vi "PassInterception.vi"(7 "Ally?":bool, 8 "error in (no error)":errorcluster, 9 "Game":refnum<class "Game.lvclass">, 10 "Point":dbl[](array[numeric]), 11 "object in":refnum<class "Utilities.lvclass">) -> (0 "error out":errorcluster, 2 "Evaluation":dbl, 3 "object out":refnum<class "Utilities.lvclass">)   [LabVIEW 2023, in "Utilities.lvclass"]
uses:
  Utilities.lvclass
  Game_class/Game.lvclass
  Game_class/Game.lvclass/Game.ctl
  Referee_class/Referee.lvclass/Referee.ctl
  Team_class/Team.lvclass/Team.ctl
  Object_class/Object.lvclass/Object.ctl
  Robot_class/Robot.lvclass/Robot.ctl
  <vilib>/Analysis/coordinate.llb/2D Cartesian Coordinate Shift (Scalar).vi
  <vilib>/Analysis/coordinate.llb/2D Cartesian Coordinate Rotation (Scalar).vi
  Robot_class/Read id.vi
  Object_class/Read position(x,y).vi
  Game_class/Read Referee.vi
  Game_class/Read EnemyRef.vi
  Game_class/Read BallRef.vi
  Game_class/Read NewParameters.vi
  Game_class/Read AllyRef.vi
  Team_class/Read RobotRef.vi
  Referee_class/Read enemy_goalie_id.vi
  Referee_class/Read our_goalie_id.vi
  Ally_class/Ally.lvclass
  Ball_class/Ball.lvclass
  Enemy_class/Enemy.lvclass
  Robot_class/Robot.lvclass
  Referee_class/Referee.lvclass
  <vilib>/Analysis/NI_AALPro.lvlib
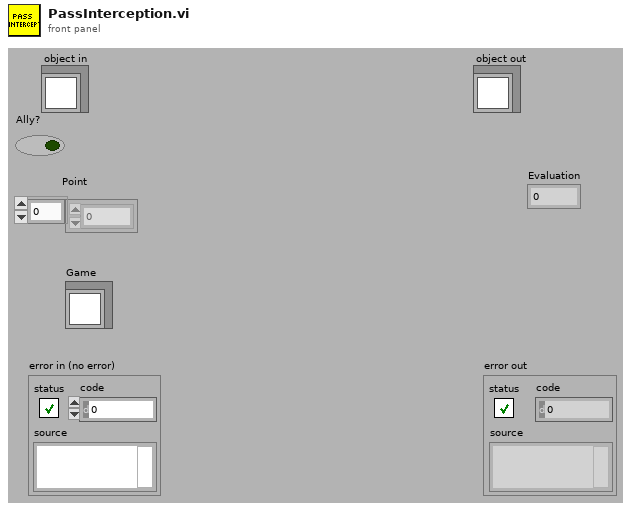
[diagram p1: front panel]
types:
  T1 = typedef "NewParameters.ctl" = cluster{"PenaltyDistance":dbl, "DistanceAttackerToBackBall":dbl, "Division":enum16{"Div B", "Div A"}, "DistanceToAvoidyEnemyRobot":dbl, "BallPlacementDistance":dbl, "DisatanceBehindBallToStealBall":dbl, "MaxDistanceToPositionKickoff":dbl, "BlockEnemyTarget":bool, "MaxStopVAng":dbl, "DistanceMarkerToEnemy":dbl, "IgnoreDribblerContact":bool, "DistanceToBeginEnemyPosession":dbl, "GoToBallWhenEnemyNotMoving":bool, "EnemyDistanceToReduceVelocity":dbl, "TurnOnEnemyDistanceToReduceVelocity":bool, "EnemyDistanceToShootOutBall":dbl, "DefenseKickBall":bool, "MoreKickToGoal? (0-0.3)":dbl, "ChipKickInEnemyField":bool, "ShootOutRobotId":dbl, "FieldLenghtDenominatorInShootOut":dbl, "AdjustPositionInBallPlacement":bool, "PowerGodPass":dbl, "VelocityAbortEnemyPos":dbl, "MaxDistToBeginPass":dbl, "MinDistToBeginPass":dbl, "VelocityInDirects":dbl, "BadDribblerIDs":i32[], "NewKickToDistanceAroundBall":dbl, "PowerAvoidColisionMarker":dbl, "DistanceToAvoidColisionMarker":dbl, "AvoidBallKick":dbl, "DistanceTryKick":dbl, "SuicideKickDIstance":dbl, "AdjustFirstKickDistance":dbl, "AvoidAimLessKick":dbl, "DistanceToAvoidyEnemyShootRobot ":dbl, "NumberOfMarkers":dbl, "PotField":bool, "PIDLateral":bool, "MinDistanceFirstKickX":dbl, "MinDistanceFirstKickY":dbl, "FractionOfDistToTouchGround\nAfterChipKick":dbl, "FractionOfKickxWhen\nComposedWithKickz":dbl, "Style":T2, "MoveInTurnState":bool, "DistFromEnemyToConsider\nMoveInTurnState":dbl, "CascadePID":bool, "TurnAroundParameters":cluster{"Radius":dbl, "Multiplier":dbl, "ChordAngle":dbl}, "SafeDriveVel":dbl, "DistanceToGoToBackBall":dbl, "minDistanceToNotFinishEnemyPossession":dbl, "OneTouchShot":cluster{"angleFactor":dbl, "maxAngle":dbl, "Attack":bool, "Defense":bool}, "OpenAngleToGoal":cluster{"minAngle":dbl, "maxAngle":dbl, "minEvaluation":dbl}, "ShotInterception":cluster{"shotSpeed":dbl, "minEnemySpeed":dbl, "maxEnemySpeed":dbl, "minEvaluation":dbl}, "AllyTeamArray":T3[], "maxDefendersNumber":i32, "Zone":cluster{"GuardPositionArray":dbl[][], "ZoneMidField":dbl[], "CenterForwardWidth":dbl}, "MinEvaluationToShoot":dbl, "PassInterception":cluster{"maxPassSpeed":dbl, "minPassSpeed":dbl, "minEnemySpeed":dbl, "chipPassDistance":dbl, "chipPassEvaluation":dbl, "minEvaluation":dbl, "maxEnemySpeed":dbl}, "PassDistance":cluster{"maxDistance":dbl, "minDistance":dbl}}
  T2 = typedef "Style.ctl" = enum16{"Insanity", "Offensive", "Defensive"}
  T3 = typedef "AllyTeam.ctl" = enum16{"Keeper", "Defender", "Attacker"}
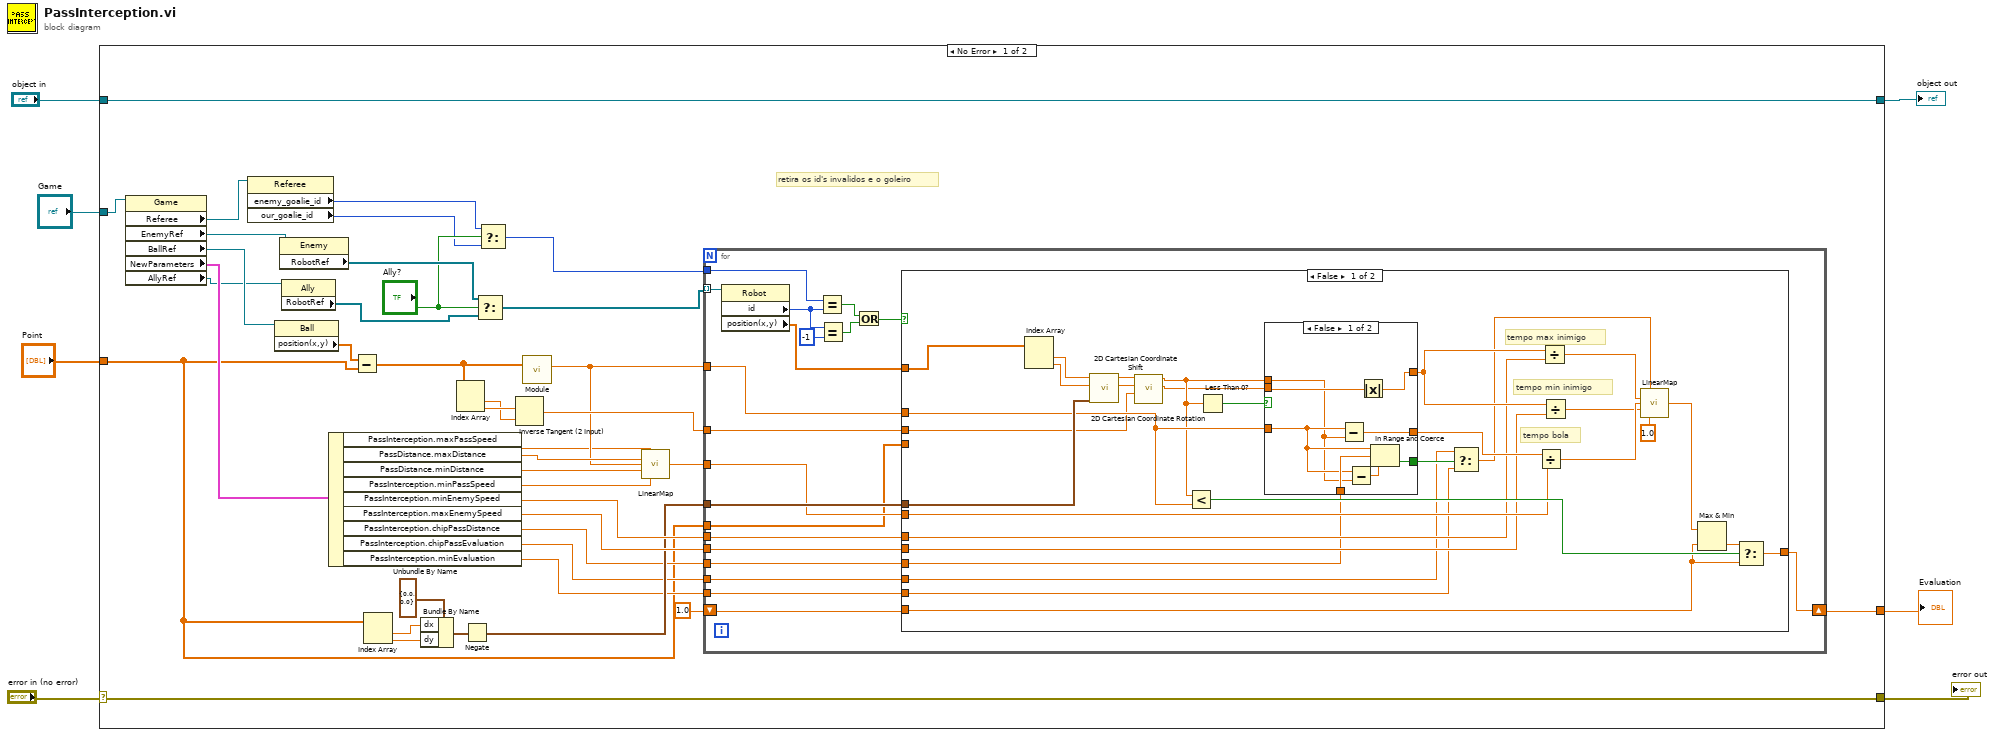
[diagram p0: block diagram]
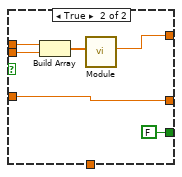
[diagram p2: hidden frame]
diagram:
  n1 = case shown="No Error" "error in (no error)" {
    selector: "error in (no error)" -> [w46 w113]
    tunnel: [w46 w113] -> w6
    tunnel: [w45 w112] -> w4
    tunnel: "object in" -> [w45 w112]
    tunnel: [w10 _] -> w3
    tunnel: "Point" -> [w9 _]
    tunnel: "Game" -> [w8 _]
    frame No Error {
      # "retira os id's invalidos e o goleiro"
      n2 = property class="Game"(reference=w8) -> ("Referee"=w43:refnum<class "Referee.lvclass">, "EnemyRef"=w44:refnum<class "Enemy.lvclass">, "BallRef"=w42:refnum<class "Ball.lvclass">, "NewParameters"=w34:T1, "AllyRef"=w12:refnum<class "Ally.lvclass">)  [unwired: 1 in, 2 out]
      n3 = property class="Referee"(reference=w43) -> ("enemy_goalie_id"=w15:i32, "our_goalie_id"=w13:i32)  [unwired: 1 in, 2 out]
      n4 = property class="Ball"(reference=w42) -> ("position(x,y)"=w19:dbl[])  [unwired: 1 in, 2 out]
      n5 = property class="Enemy"(reference=w44) -> ("RobotRef"=w18:refnum<class "Robot.lvclass">[])  [unwired: 1 in, 2 out]
      n6 = property class="Ally"(reference=w12) -> ("RobotRef"=w11:refnum<class "Robot.lvclass">[])  [unwired: 1 in, 2 out]
      n7 = Unbundle By Name(w34) -> ("PassInterception.maxPassSpeed"=w27:dbl, "PassDistance.maxDistance"=w33:dbl, "PassDistance.minDistance"=w32:dbl, "PassInterception.minPassSpeed"=w28:dbl, "PassInterception.minEnemySpeed"=w26:dbl, "PassInterception.maxEnemySpeed"=w25:dbl, "PassInterception.chipPassDistance"=w22:dbl, "PassInterception.chipPassEvaluation"=w21:dbl, "PassInterception.minEvaluation"=w20:dbl)
      n8 = Subtract(x=w19, y=w9) -> (x-y=w35:dbl[])
      n9 = Index Array(array=w9) -> (element #1=w37:dbl, element #2=w36:dbl)  [unwired: 2 in]
      n10 = Bundle By Name(cluster=cluster{"dx":dbl, "dy":dbl} {"dx"=0.0, "dy"=0.0} ("shift"), "dx"=w37, "dy"=w36) -> (w24:cluster{"dx":dbl, "dy":dbl})
      n11 = Index Array(array=w35) -> (element #1=w40:dbl, element #2=w41:dbl)  [unwired: 2 in]
      n12 = Negate(x=w24) -> (-x=w23:cluster{"dx":dbl, "dy":dbl})
      n13 = Select(t=w18, s="Ally?", f=w11) -> (s? t:f=w17:refnum<class "Robot.lvclass">[])
      n14 = Select(t=w15, s="Ally?", f=w13) -> (s? t:f=w14:i32)
      n15 = Inverse Tangent (2 Input)(1:w40, 2:w41) -> (0:w39:dbl)
      n16 = call "Module.vi"("2D vector"=w35) -> ("Modulo"=w31:dbl)  [unwired: 8 in, 2 out]
      n17 = call "LinearMap.vi"("MaxY"=w27, "MaxX"=w33, "X"=w31, "MinX"=w32, "MinY"=w28) -> ("Y"=w30:dbl)  [unwired: 8 in, 2 out]
      n18 = for {
        tunnel: w17 -> [w65] mode=indexing
        tunnel: w14 -> [w47]
        tunnel: w39 -> [w60]
        tunnel: w23 -> [w58]
        tunnel: w31 -> [w57]
        tunnel: w30 -> [w56]
        shift-right: [w54] -> w10
        shift-left: 1.0 ("Numeric") -> [w55]
        tunnel: w9 -> [w53]
        tunnel: w26 -> [w52]
        tunnel: w25 -> [w51]
        tunnel: w22 -> [w50]
        tunnel: w21 -> [w49]
        tunnel: w20 -> [w48]
        n19 = property class="Robot"(reference=w65) -> ("id"=w64:i32, "position(x,y)"=w59:dbl[])  [unwired: 1 in, 2 out]
        n20 = Equal?(x=w47, y=w64) -> (x = y?=w62:bool)
        n21 = Equal?(x=w64, y=-1) -> (x = y?=w61:bool)
        n22 = Or(x=w62, y=w61) -> (x .or. y?=w66:bool)
        n23 = case shown="False" w66 {
          tunnel: w60 -> [w78 _]
          tunnel: w59 -> [w92 _]
          tunnel: w58 -> [w96 _]
          tunnel: w57 -> [w87 _]
          tunnel: w56 -> [w88 _]
          tunnel: w55 -> [w79 w111]
          tunnel: [w93 w111] -> w54
          tunnel: w53 -> [_ _]
          tunnel: w52 -> [w85 _]
          tunnel: w51 -> [w84 _]
          tunnel: w50 -> [w71 _]
          tunnel: w49 -> [w68 _]
          tunnel: w48 -> [w67 _]
          frame False {
            # "tempo bola"
            # "tempo min inimigo"
            # "tempo max inimigo"
            n24 = Index Array(array=w92) -> (element #1=w77:dbl, element #2=w76:dbl)  [unwired: 2 in]
            n25 = call-poly <vilib>:"2D Cartesian Coordinate Shift.vi"("shift"=w96, "y"=w76, "x"=w77) -> ("y out"=w74:dbl, "x out"=w75:dbl)  [unwired: 6 in, 1 out]
            n26 = call-poly <vilib>:"2D Cartesian Coordinate Rotation.vi"("theta"=w78, "y"=w74, "x"=w75) -> ("y out"=w72:dbl, "x out"=w73:dbl)  [unwired: 6 in, 1 out]
            n27 = Less?(x=w73, y=w87) -> (x < y?=w94:bool)
            n28 = Less Than 0?(x=w73) -> (x < 0?=w95:bool)
            n29 = case shown="False" w95 {
              tunnel: w73 -> [w97 w108]
              tunnel: w72 -> [w103 w106]
              tunnel: [w102 w110] -> w89
              tunnel: w87 -> [w99 w109]
              tunnel: [w104 w109] -> w86
              tunnel: w71 -> [w100 _]
              tunnel: [w98 FALSE] -> w69
              frame False {
                n30 = Subtract(x=w99, y=w97) -> (x-y=w104:dbl)
                n31 = Subtract(x=w99, y=w97) -> (x-y=w101:dbl)
                n32 = Absolute Value(x=w103) -> (abs(x)=w102:dbl)
                n33 = In Range and Coerce(upper limit=w99, x=w100, lower limit=w101) -> (In Range?=w98:bool)  [unwired: 1 out]
              }
              frame True {
                n34 = Build Array(w108, w106) -> (w107:dbl[])
                n35 = call "Module.vi"("2D vector"=w107) -> ("Modulo"=w110:dbl)  [unwired: 8 in, 2 out]
              }
            }
            n36 = Select(t=w68, s=w69, f=w67) -> (s? t:f=w70:dbl)
            n37 = Divide(x=w86, y=w88) -> (x/y=w91:dbl)
            n38 = Divide(x=w89, y=w85) -> (x/y=w83:dbl)
            n39 = Divide(x=w89, y=w84) -> (x/y=w82:dbl)
            n40 = call "LinearMap.vi"("MaxY"=w70, "MaxX"=w83, "X"=w91, "MinX"=w82, "MinY"=1.0) -> ("Y"=w81:dbl)  [unwired: 8 in, 2 out]
            n41 = Max & Min(x=w81, y=w79) -> (min(x,y)=w80:dbl)  [unwired: 1 out]
            n42 = Select(t=w80, s=w94, f=w79) -> (s? t:f=w93:dbl)
          }
          frame True {
          }
        }
      }
    }
    frame Error {
    }
  }
  "error out" <- w6
  "object out" <- w4
  "Evaluation" <- w3
